vi "Reporter.vi"(8 "error in (no error)":errorcluster caption="エラー入力（エラーなし）", 9 "Assertion Result":T1, 10 "Operation":T2) -> (0 "error out":errorcluster caption="エラー出力")   [LabVIEW 2014, in "Monitor.lvlib" / "Testing.lvlib"]
uses:
  Testing.lvlib
  AssertionResult.ctl
  ReporterOperation.ctl
panel:
  out "all passed":bool
  out "Results":T1[](array[typedef])
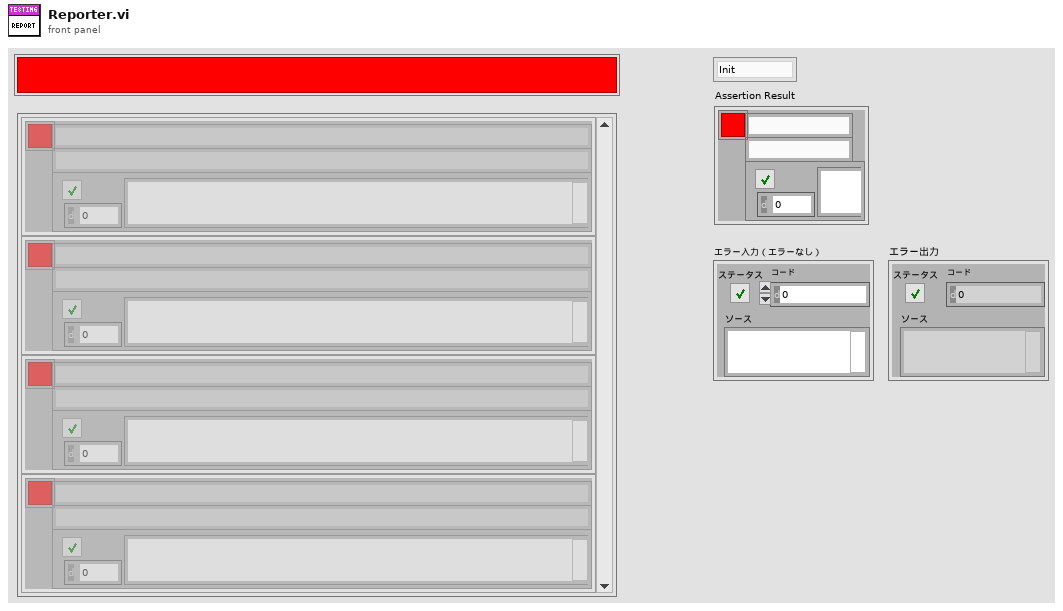
[diagram p1: front panel]
types:
  T1 = typedef "Monitor.lvlib/Testing.lvlib/AssertionResult.ctl" = cluster{"VI Name":string, "Comment":string, "Error":errorcluster, "Pass":bool}
  T2 = typedef "Monitor.lvlib/Testing.lvlib/ReporterOperation.ctl" = enum16{"Init", "Append"}
  T3 = enum32{"Invalid", "Standard", "Closed", "Hidden", "Minimized", "Maximized"}
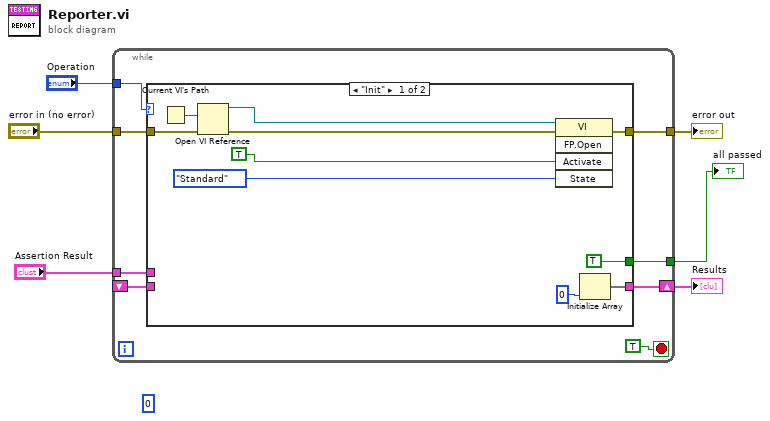
[diagram p0: block diagram]
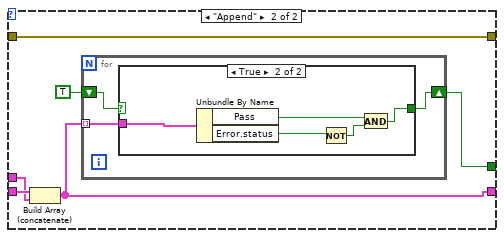
[diagram p2: hidden frame]
diagram:
  (unwired) 0
  n1 = while {
    tunnel: "Operation" -> [w13]
    shift-right: [w11] -> w3
    shift-left: _ -> [w12]
    tunnel: "error in (no error)" -> [w10]
    tunnel: [w9] -> w4
    tunnel: "Assertion Result" -> [w8]
    tunnel: [w7] -> w1
    stop <- TRUE stop-if-true
    n2 = case shown="\"Init\"" w13 {
      tunnel: w12 -> [_ w29]
      tunnel: [w23 w26] -> w11
      tunnel: w10 -> [w19 w30]
      tunnel: [w18 w30] -> w9
      tunnel: w8 -> [_ w28]
      tunnel: [TRUE ("all passed") w25] -> w7
      frame "Init" {
        n3 = Current VI's Path() -> (path=w22:path)
        n4 = Open VI Reference(vi path=w22, error in (no error)=w19) -> (vi reference=w21:refnum<vi>, error out=w20:errorcluster)  [unwired: 4 in]
        n5 = invoke class="VI" method="FP.Open"(reference=w21, error in=w20, "Activate"=TRUE ("アクティブ化?"), "State"=T3."Standard" ("状態")) -> (error out=w18:errorcluster)  [unwired: 1 in, 4 out]
        n6 = Initialize Array(0 ("次元サイズ")) -> (w23:void[])  [unwired: 1 in]
      }
      frame "Append" {
        n7 = Build Array (concatenate)(w29, w28) -> (w26:T1[])
        n8 = for {
          shift-right: [w32] -> w25
          shift-left: TRUE -> [w33]
          tunnel: w26 -> [w31] mode=indexing
          n9 = case shown="TRUE" w33 {
            selector: w33 -> [w34 _]
            tunnel: [w34 w35] -> w32
            tunnel: w31 -> [_ w39]
            frame False {
            }
            frame True {
              n10 = Unbundle By Name(w39) -> ("Pass"=w37:bool, "Error.status"=w38:bool)
              n11 = Not(x=w38) -> (.not. x?=w36:bool)
              n12 = And(x=w37, y=w36) -> (x .and. y?=w35:bool)
            }
          }
        }
      }
    }
  }
  "Results" <- w3
  "all passed" <- w1
  "error out" <- w4
